vi "PantherLAB_Log - Convert DQMH Event.vi"(6 "New Event Type":T1, 9 "New Broadcast Name":string, 10 "Event Info (Converted)":T2={"Event VI Path"=path "", "Argument Path"=path "", "Wait Argument Path"=path "", "Event Arg Owner"=-1, "Event Name"="", "Type"=enum."Request"}, 11 "Module Info":T4) -> (0 "error out":errorcluster)   [LabVIEW 2016]
doc: "_____\nCreated using DQMH Framework: Event Scripter 7.1.0.1450."
uses:
  <vilib>/Delacor/Delacor QMH/Libraries/_Scripting Support/Module Info--cluster.ctl
  <vilib>/Delacor/Delacor QMH/Libraries/_Scripting Support/Module Type--enum.ctl
  <vilib>/Delacor/Delacor QMH/Libraries/_Scripting Support/Event Info (Existing)--cluster.ctl
  Program Files (x86)/National Instruments/LabVIEW 2016/project/Delacor/DQMH/_DQMH Remove Event/Event Type (All Permutations)--enum.ctl
  <vilib>/Delacor/Delacor QMH/Libraries/_Scripting Support/Event Type (Convert)--enum.ctl
  PantherLAB Scripting Hooks/PantherLAB_Log.lvlib
  <vilib>/Delacor/Delacor QMH/Libraries/_Scripting Support/dqmh_lib_DQMH Scripting Support.lvlib
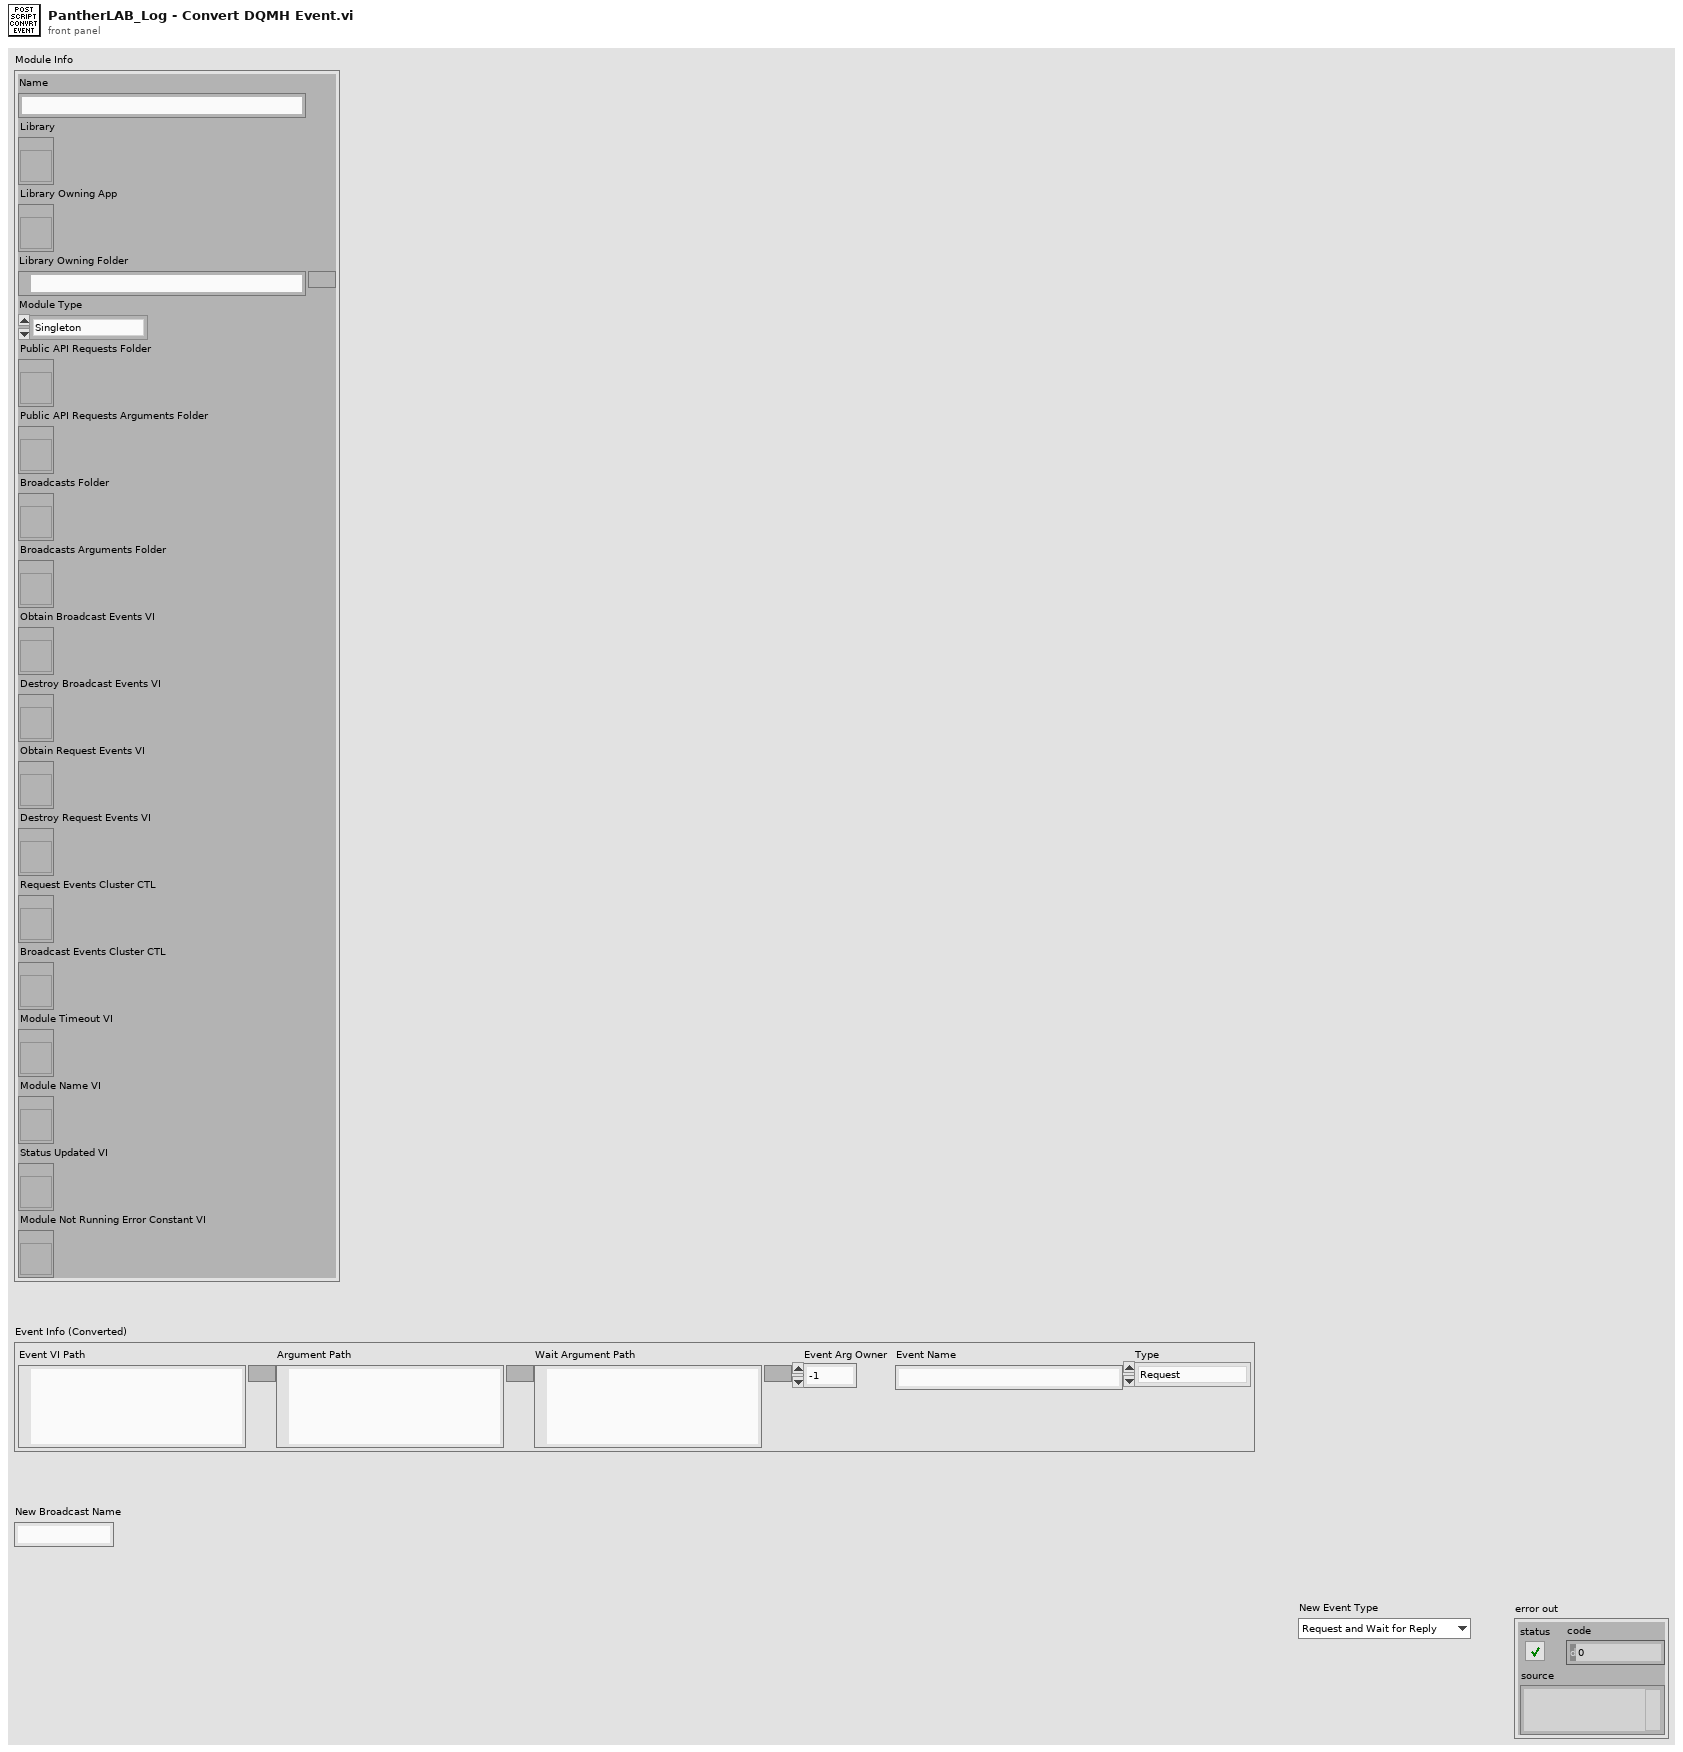
[diagram p1: front panel]
types:
  T1 = typedef "dqmh_lib_DQMH Scripting Support.lvlib/Event Type (Convert)--enum.ctl" = enum16{"Request and Wait for Reply", "Round Trip"}
  T2 = typedef "dqmh_lib_DQMH Scripting Support.lvlib/Event Info (Existing)--cluster.ctl" = cluster{"Event VI Path":path, "Argument Path":path, "Wait Argument Path":path, "Event Arg Owner":i32, "Event Name":string, "Type":T3}
  T3 = typedef "dqmh_lib_DQMH Scripting Support.lvlib/Event Type (All Permutations)--enum.ctl" = enum16{"Request", "Broadcast", "Both", "Request (no Wait)", "Request and Wait", "Request (Private)", "Request (Local Instance)"}
  T4 = typedef "dqmh_lib_DQMH Scripting Support.lvlib/Module Info--cluster.ctl" = cluster{"Name":string, "Library":refnum<vi>, "Library Owning App":refnum<vi>, "Library Owning Folder":path, "Module Type":T5, "Public API Requests Folder":refnum<vi>, "Public API Requests Arguments Folder":refnum<vi>, "Broadcasts Folder":refnum<vi>, "Broadcasts Arguments Folder":refnum<vi>, "Obtain Broadcast Events VI":refnum<vi>, "Destroy Broadcast Events VI":refnum<vi>, "Obtain Request Events VI":refnum<vi>, "Destroy Request Events VI":refnum<vi>, "Request Events Cluster CTL":refnum<vi>, "Broadcast Events Cluster CTL":refnum<vi>, "Module Timeout VI":refnum<vi>, "Module Name VI":refnum<vi>, "Status Updated VI":refnum<vi>, "Module Not Running Error Constant VI":refnum<vi>}
  T5 = typedef "dqmh_lib_DQMH Scripting Support.lvlib/Module Type--enum.ctl" = enum16{"Singleton", "Cloneable"}
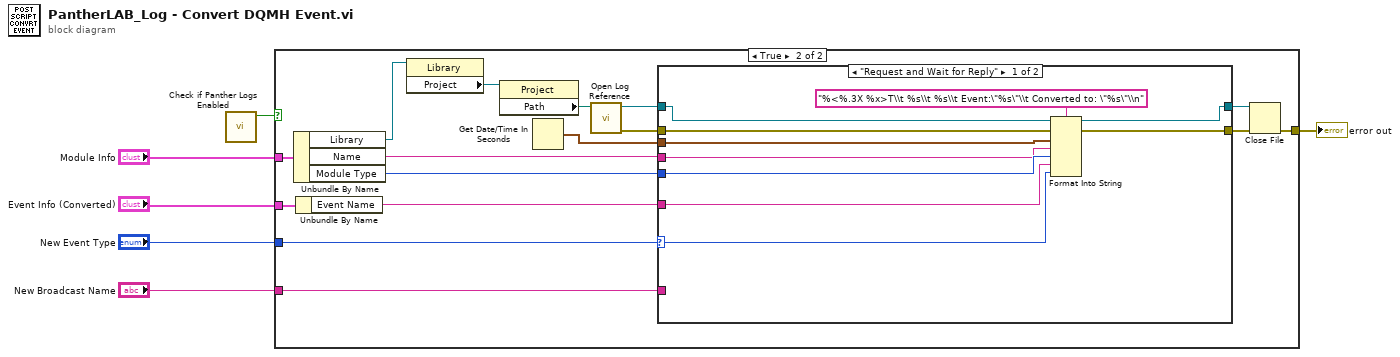
[diagram p0: block diagram]
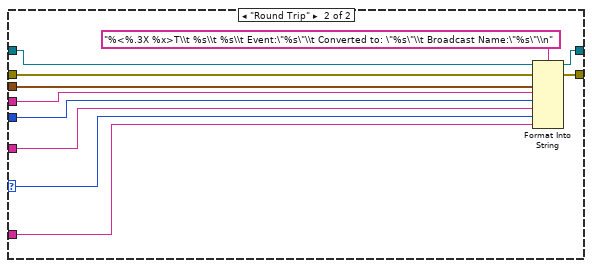
[diagram p3: hidden frame]
diagram:
  n1 = call "Check if Panther Logs Enabled.vi"() -> ("PantherLogs Enabled?"=w5:bool)  [unwired: 11 in]
  n2 = case shown="True" w5 {
    tunnel: [_ w20] -> w6
    tunnel: "Module Info" -> [_ w19]
    tunnel: "Event Info (Converted)" -> [_ w16]
    tunnel: "New Broadcast Name" -> [_ w8]
    tunnel: "New Event Type" -> [_ w9]
    frame False {
    }
    frame True {
      n3 = Unbundle By Name(w19) -> ("Library"=w18:refnum<vi>, "Name"=w13:string, "Module Type"=w12:T5)
      n4 = Unbundle By Name(w16) -> ("Event Name"=w7:string)
      n5 = property class="Library"(reference=w18) -> ("Project"=w17:refnum<vi>)  [unwired: 1 in, 2 out]
      n6 = property class="Project"(reference=w17) -> ("Path"=w10:path)  [unwired: 1 in, 2 out]
      n7 = Get Date/Time In Seconds() -> (seconds since 1Jan1904=w11:timestamp)
      n8 = call "Open Log Reference.vi"("Project Path"=w10) -> ("error out"=w22:errorcluster, "File Reference"=w15:refnum<file>)  [unwired: 9 in]
      n9 = case shown="\"Request and Wait for Reply\"" w9 {
        selector: w9 -> [w24 w35]
        tunnel: w15 -> [w30 w41]
        tunnel: w22 -> [w32 w43]
        tunnel: [w29 w40] -> w14
        tunnel: [w31 w42] -> w21
        tunnel: w13 -> [w27 w38]
        tunnel: w12 -> [w28 w39]
        tunnel: w11 -> [w26 w37]
        tunnel: w8 -> [_ w33]
        tunnel: w7 -> [w25 w36]
        frame "Request and Wait for Reply" {
          n10 = Format Into String(format string="%<%.3X %x>T\\t %s\\t %s\\t Event:\"%s\"\\t Converted to: \"%s\"\\n", initial string=w30, error in=w32, w26, w27, w28, w25, w24) -> (resulting string=w29:refnum<file>, error out=w31:errorcluster)
        }
        frame "Round Trip" {
          n11 = Format Into String(format string="%<%.3X %x>T\\t %s\\t %s\\t Event:\"%s\"\\t Converted to: \"%s\"\\t Broadcast Name:\"%s\"\\n", initial string=w41, error in=w43, w37, w38, w39, w36, w35, w33) -> (resulting string=w40:refnum<file>, error out=w42:errorcluster)
        }
      }
      n12 = Close File(refnum=w14, error in=w21) -> (error out=w20:errorcluster)  [unwired: 1 out]
    }
  }
  "error out" <- w6
